vi "WriteFromTDMStoFIFO_EDVR.vi"(4 "Previewed Channel":T1, 6 "Samples per Write":u32, 7 "Infinite Generation":bool, 8 "error in (no error)":errorcluster, 9 "Queue in":refnum<queue>, 10 "HSS refnum in":refnum<k20>, 11 "TDMS read controls in":T2[](array[typedef])) -> (0 "error out":errorcluster, 2 "read process finished?":bool, 3 "TDMS read controls out":T2[](array[typedef]), 5 "Channels Running?":bool[](array[boolean]))   [LabVIEW 2018]
uses:
  TypeDefs/TDMS read.ctl
  TDMS Raw to Channels/Previewed Channel - Enum.ctl
  <vilib>/Utility/error.llb/Error Cluster From Error Code.vi
  <vilib>/rvi/errors/niLvFpgaAdjustHostInterfaceError.vi
  <vilib>/rvi/interface/nirviMethod/nirviMethod.xnode
  <vilib>/FPGAPlugInAG/Dynamic/niLvFpga_AcquireWriteRegionFifo_Dynamic.vi
  <vilib>/rvi/errors/niLvFpgaMergeErrorWithErrorCode.vi
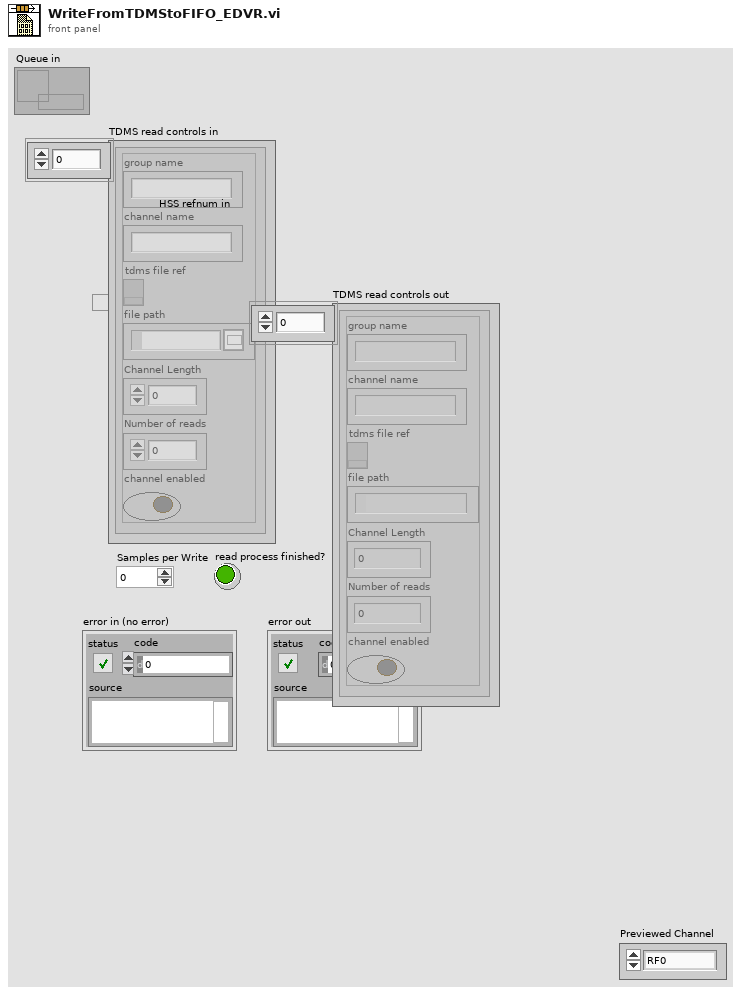
[diagram p1: front panel]
types:
  T1 = typedef "Previewed Channel - Enum.ctl" = enum16{"RF0", "RF1"}
  T2 = typedef "TDMS read.ctl" = cluster{"group name":string, "channel name":string, "tdms file ref":refnum<k34>, "file path":path, "Channel Length":i64, "Number of reads":i64, "channel enabled":bool}
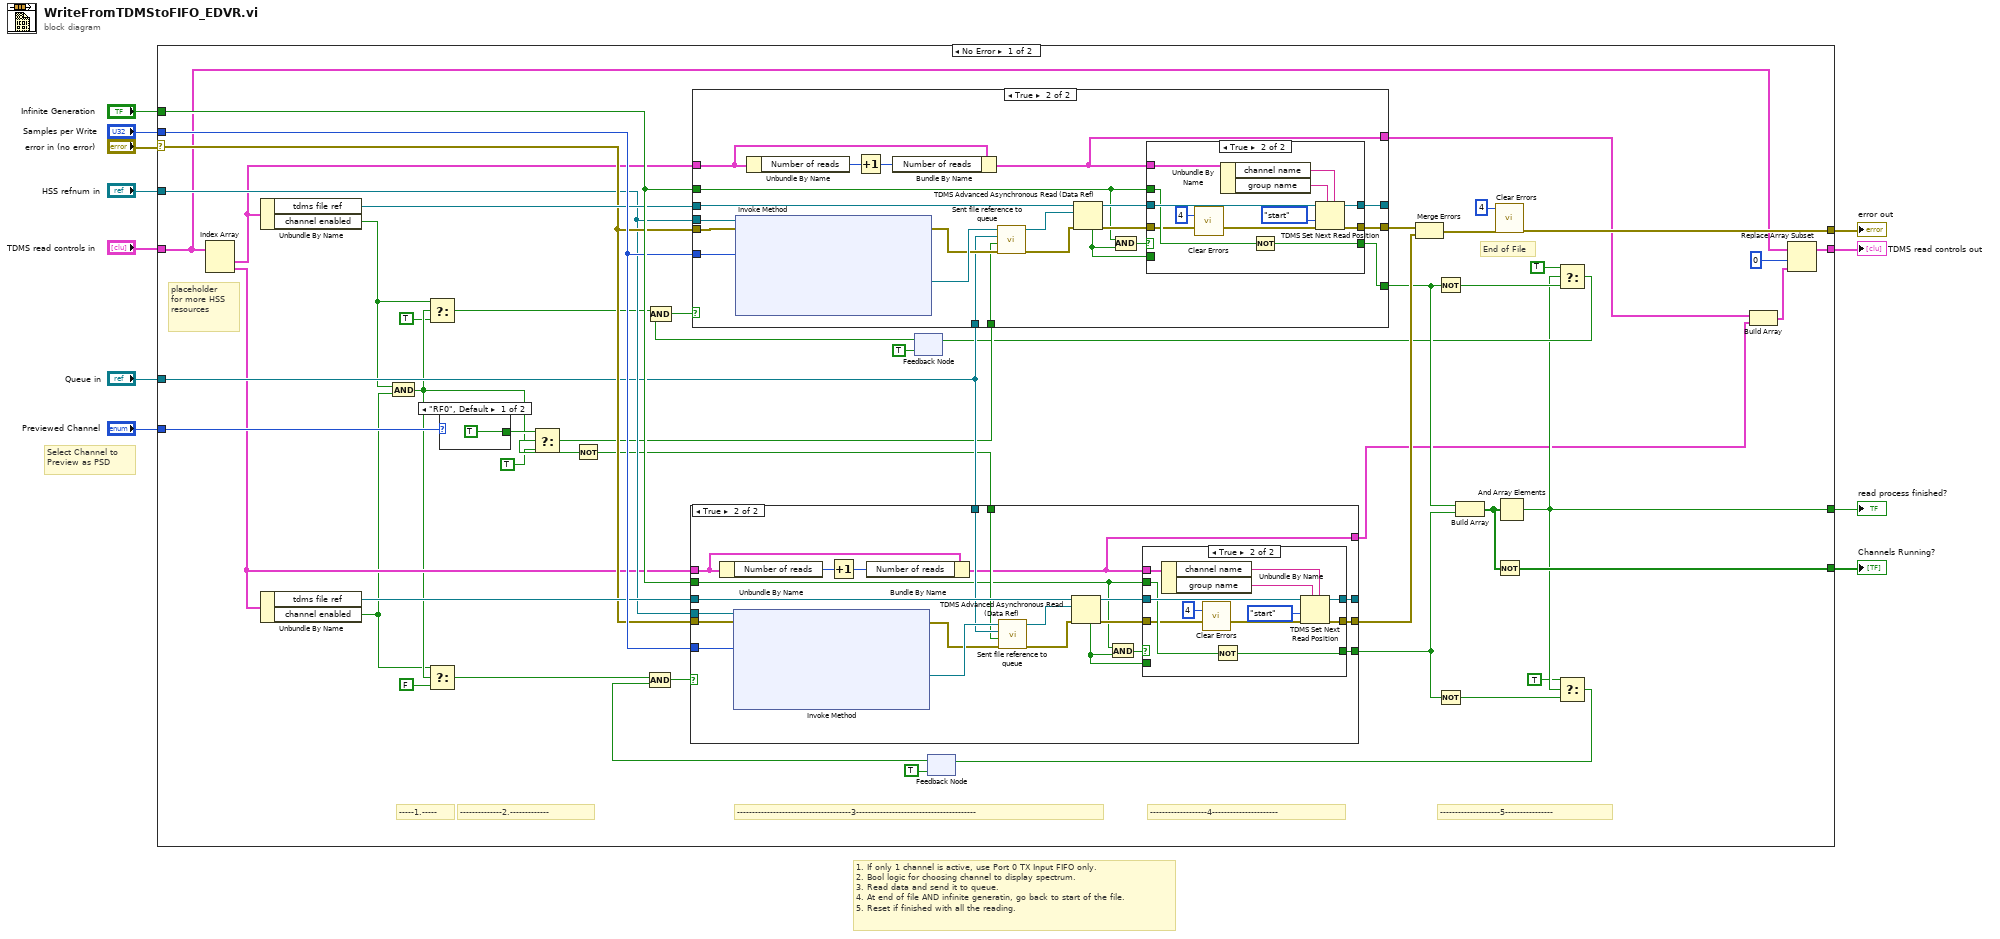
[diagram p0: block diagram]
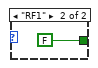
[diagram p2: hidden frame]
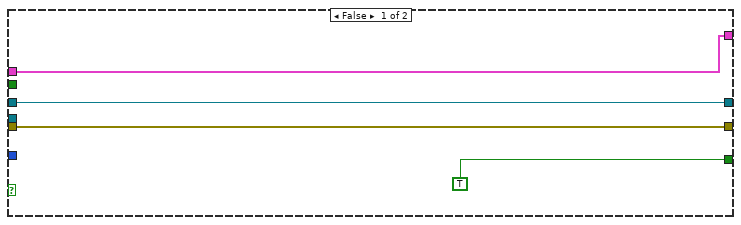
[diagram p3: hidden frame]
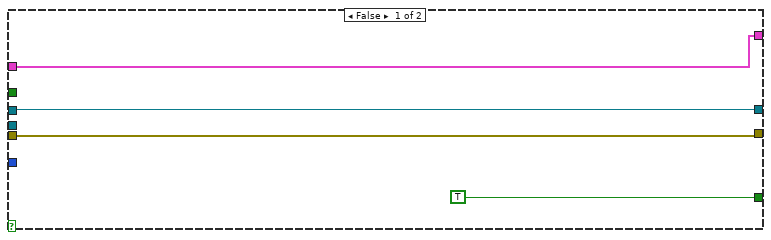
[diagram p5: hidden frame]
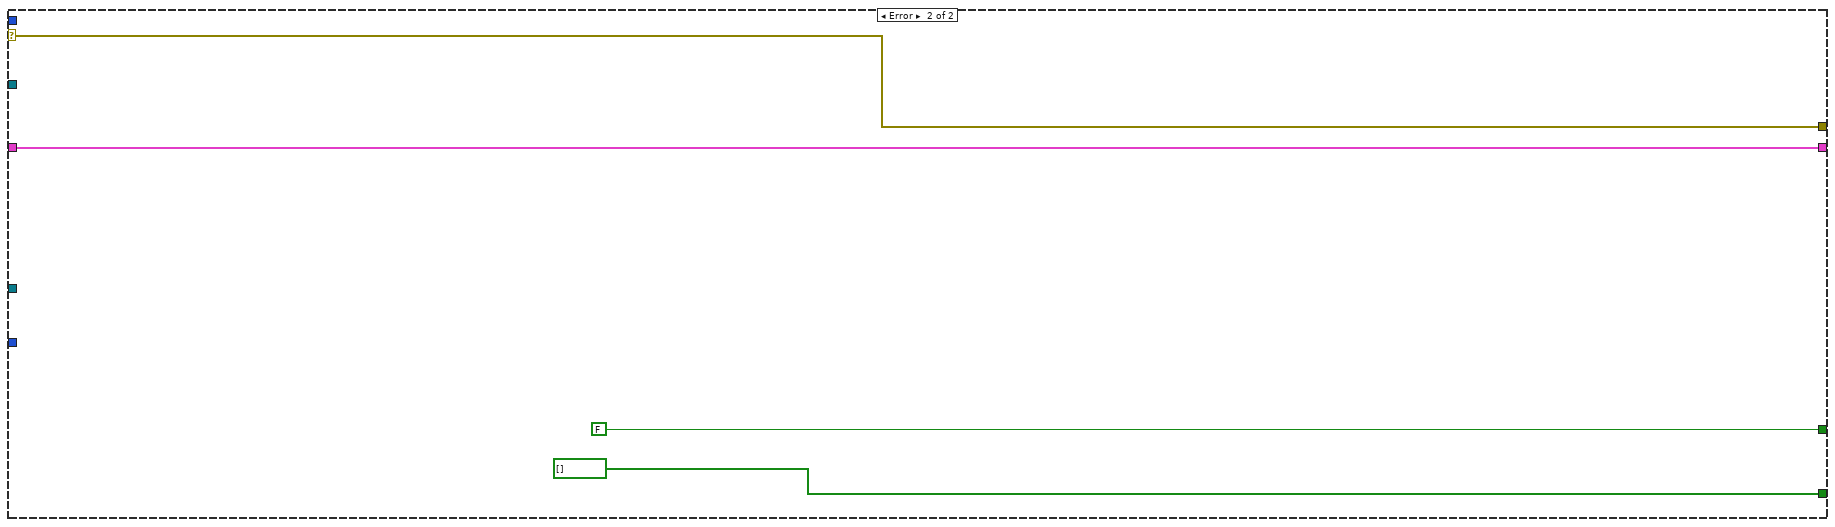
[diagram p7: hidden frame]
diagram:
  # "1. If only 1 channel is active, use Port 0 TX Input FIFO only.\n2. Bool logic for choosing channel to display spectrum.\n3. Read data and send it to queue.\n4. At end of file AND infinite generatin, go back to start of the file.\n5. Reset if finished with all the reading."
  # "Select Channel to \nPreview as PSD"
  n1 = case shown="No Error" "error in (no error)" {
    selector: "error in (no error)" -> [w45 w148]
    tunnel: [w60 w148] -> w11
    tunnel: [w36 bool[] []] -> w10
    tunnel: "Infinite Generation" -> [w49 _]
    tunnel: [w18 FALSE] -> w8
    tunnel: "Samples per Write" -> [w48 _]
    tunnel: "HSS refnum in" -> [w44 _]
    tunnel: "TDMS read controls in" -> [w34 w145]
    tunnel: "Queue in" -> [w43 _]
    tunnel: "Previewed Channel" -> [w42 _]
    tunnel: [w31 w145] -> w1
    frame No Error {
      # "--------------------5----------------"
      # "-------------------4----------------------"
      # "--------------------------------------3----------------------------------------"
      # "-----1.-----"
      # "--------------2.-------------"
      # "placeholder for more HSS resources"
      # "End of File"
      n2 = Index Array(array=w34) -> (element #1=w40:T2, element #2=w39:T2)  [unwired: 2 in]
      n3 = Unbundle By Name(w40) -> ("tdms file ref"=w47:refnum<k34>, "channel enabled"=w28:bool)
      n4 = Unbundle By Name(w39) -> ("tdms file ref"=w46:refnum<k34>, "channel enabled"=w26:bool)
      n5 = And(x=w28, y=w26) -> (x .and. y?=w27:bool)
      n6 = Select(t=w28, s=w27, f=TRUE) -> (s? t:f=w24:bool)
      n7 = Select(t=w26, s=w27, f=FALSE) -> (s? t:f=w22:bool)
      n8 = case shown="\"RF0\", Default" w42 {
        tunnel: [TRUE FALSE] -> w41
        frame "RF0", Default {
        }
        frame "RF1" {
        }
      }
      n9 = Select(t=w41, s=w27, f=TRUE) -> (s? t:f=w30:bool)
      n10 = Not(x=w30) -> (.not. x?=w29:bool)
      n11 = feedback #1(TRUE ("read process finished?")) -> (w51:bool)
      n12 = Compound Arithmetic op=AND(w24, w51) -> (w50:bool)
      n13 = case shown="True" w50 {
        tunnel: w44 -> [_ w129]
        tunnel: [w107 w123] -> w58
        tunnel: w45 -> [w107 w128]
        tunnel: w48 -> [_ w127]
        tunnel: w47 -> [w104 w126]
        tunnel: [TRUE w112] -> w38
        tunnel: w49 -> [_ w110]
        tunnel: w40 -> [w105 w115]
        tunnel: w43 -> [_ w118]
        tunnel: w30 -> [_ w117]
        tunnel: [w105 w113] -> w13
        tunnel: [w104 w108] -> _
        frame False {
        }
        frame True {
          n14 = xnode "Invoke Method"("FPGA VI Reference In"=w129, "error in"=w128, "Number of Elements"=w127) -> ("error out"=w119:errorcluster, "Write Region Reference"=w122:refnum<data-value>)  [unwired: 1 in, 3 out]
          n15 = Unbundle By Name(w115) -> ("Number of reads"=w116:i64)
          n16 = Increment(x=w116) -> (x+1=w114:i64)
          n17 = Bundle By Name(cluster=w115, "Number of reads"=w114) -> (w113:T2)
          n18 = call "Sent file reference to queue.vi"("error in (no error)"=w119, "Send?"=w117, "Queue in"=w118, "Write Region Reference"=w122) -> ("error out"=w120:errorcluster, "Data Value Reference out"=w121:refnum<data-value>)  [unwired: 6 in]
          n19 = TDMS Advanced Asynchronous Read (Data Ref)(8:w120, 10:w121, 11:w126) -> (0:w124:errorcluster, 3:w125:refnum<k34>, 4:w109:bool)  [unwired: 1 in]
          n20 = And(x=w110, y=w109) -> (x .and. y?=w111:bool)
          n21 = case shown="True" w111 {
            tunnel: w125 -> [w130 w143]
            tunnel: w124 -> [w132 w134]
            tunnel: [w132 w142] -> w123
            tunnel: w113 -> [_ w141]
            tunnel: [w131 w137] -> w112
            tunnel: w110 -> [_ w138]
            tunnel: w109 -> [w131 _]
            tunnel: [w130 w133] -> w108
            frame False {
            }
            frame True {
              n22 = call <vilib>:"Clear Errors.vi"("error in (no error)"=w134, "specific error code to clear (0: all)"=4) -> ("error out"=w135:errorcluster)  [unwired: 4 in, 1 out]
              n23 = Unbundle By Name(w141) -> ("channel name"=w140:string, "group name"=w139:string)
              n24 = Not(x=w138) -> (.not. x?=w137:bool)
              n25 = TDMS Set Next Read Position(5:w140, 7:w139, 8:w135, 9:enum16{"start", "end"}."start" ("from (0: start)"), 11:w143) -> (0:w142:errorcluster, 3:w133:refnum<k34>)  [unwired: 1 in]
            }
          }
        }
      }
      n26 = feedback #2(TRUE ("read process finished?")) -> (w53:bool)
      n27 = Compound Arithmetic op=AND(w22, w53) -> (w52:bool)
      n28 = case shown="True" w52 {
        tunnel: [w66 w83] -> w56
        tunnel: w44 -> [_ w88]
        tunnel: w46 -> [w63 w87]
        tunnel: w48 -> [_ w86]
        tunnel: w45 -> [w66 w85]
        tunnel: [TRUE w71] -> w35
        tunnel: w49 -> [_ w70]
        tunnel: w39 -> [w64 w73]
        tunnel: w43 -> [_ w77]
        tunnel: w29 -> [_ w76]
        tunnel: [w64 w72] -> w12
        tunnel: [w63 w67] -> _
        frame False {
        }
        frame True {
          n29 = Unbundle By Name(w73) -> ("Number of reads"=w75:i64)
          n30 = xnode "Invoke Method"("FPGA VI Reference In"=w88, "error in"=w85, "Number of Elements"=w86) -> ("error out"=w79:errorcluster, "Write Region Reference"=w80:refnum<data-value>)  [unwired: 1 in, 3 out]
          n31 = Increment(x=w75) -> (x+1=w74:i64)
          n32 = Bundle By Name(cluster=w73, "Number of reads"=w74) -> (w72:T2)
          n33 = call "Sent file reference to queue.vi"("error in (no error)"=w79, "Send?"=w76, "Queue in"=w77, "Write Region Reference"=w80) -> ("error out"=w78:errorcluster, "Data Value Reference out"=w81:refnum<data-value>)  [unwired: 6 in]
          n34 = TDMS Advanced Asynchronous Read (Data Ref)(8:w78, 10:w81, 11:w87) -> (0:w84:errorcluster, 3:w82:refnum<k34>, 4:w68:bool)  [unwired: 1 in]
          n35 = And(x=w70, y=w68) -> (x .and. y?=w69:bool)
          n36 = case shown="True" w69 {
            tunnel: w82 -> [w89 w102]
            tunnel: w84 -> [w91 w95]
            tunnel: [w91 w101] -> w83
            tunnel: w72 -> [_ w100]
            tunnel: [w90 w96] -> w71
            tunnel: w70 -> [_ w97]
            tunnel: w68 -> [w90 _]
            tunnel: [w89 w92] -> w67
            frame False {
            }
            frame True {
              n37 = Unbundle By Name(w100) -> ("channel name"=w99:string, "group name"=w98:string)
              n38 = call <vilib>:"Clear Errors.vi"("error in (no error)"=w95, "specific error code to clear (0: all)"=4) -> ("error out"=w94:errorcluster)  [unwired: 4 in, 1 out]
              n39 = Not(x=w97) -> (.not. x?=w96:bool)
              n40 = TDMS Set Next Read Position(5:w99, 7:w98, 8:w94, 9:enum16{"start", "end"}."start" ("from (0: start)"), 11:w102) -> (0:w101:errorcluster, 3:w92:refnum<k34>)  [unwired: 1 in]
            }
          }
        }
      }
      n41 = Merge Errors(w58, w56) -> (w57:errorcluster)
      n42 = Not(x=w38) -> (.not. x?=w20:bool)
      n43 = Not(x=w35) -> (.not. x?=w17:bool)
      n44 = Build Array(w38, w35) -> (w37:bool[])
      n45 = call <vilib>:"Clear Errors.vi"("error in (no error)"=w57, "specific error code to clear (0: all)"=4) -> ("error out"=w60:errorcluster)  [unwired: 4 in, 1 out]
      n46 = Not(x=w37) -> (.not. x?=w36:bool[])
      n47 = And Array Elements(Boolean array=w37) -> (logical AND=w18:bool)
      n48 = Select(t=TRUE, s=w18, f=w20) -> (s? t:f=w19:bool)
      n49 = feedback-in #1(w19) -> ()
      n50 = Select(t=TRUE, s=w18, f=w17) -> (s? t:f=w16:bool)
      n51 = feedback-in #2(w16) -> ()
      n52 = Build Array(w13, w12) -> (w33:T2[])
      n53 = Replace Array Subset(array=w34, new element=w33, index=0) -> (w31:T2[])
    }
    frame Error {
    }
  }
  "error out" <- w11
  "read process finished?" <- w8
  "Channels Running?" <- w10
  "TDMS read controls out" <- w1
